vi "wifiSim.vi"(8 "error in (no error)":errorcluster, 10 "REPL":string, 11 "Server":path) -> ()   [LabVIEW 2020]
panel:
  out "concatenated string":string
  out "x .and. y?":bool
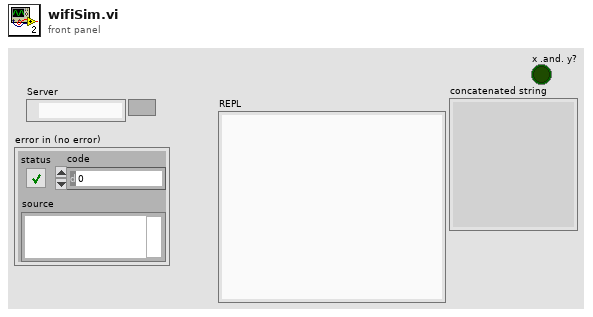
[diagram p1: front panel]
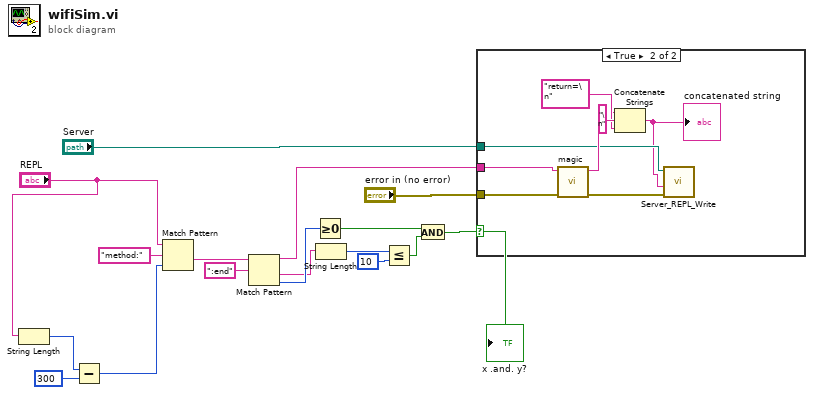
[diagram p0: block diagram]
diagram:
  n1 = String Length(string="REPL") -> (length=w3:i32)
  n2 = Subtract(x=w3, y=300) -> (x-y=w1:i32)
  n3 = Match Pattern(string="REPL", regular expression="method:" ("First"), offset (0)=w1) -> (after substring=w13:string)  [unwired: 3 out]
  n4 = Match Pattern(string=w13, regular expression=":end" ("Last")) -> (before substring=w15:string, after substring=w10:string, offset past match=w14:i32)  [unwired: 1 in, 1 out]
  n5 = Greater Or Equal To 0?(x=w14) -> (x >= 0?=w6:bool)
  n6 = String Length(string=w10) -> (length=w9:i32)
  n7 = Less Or Equal?(x=w9, y=10) -> (x <= y?=w7:bool)
  n8 = And(x=w6, y=w7) -> (x .and. y?=w5:bool)
  "x .and. y?" <- w5
  n9 = case shown="True" w5 {
    tunnel: w15 -> [_ w25]
    tunnel: "error in (no error)" -> [_ w24]
    tunnel: "Server" -> [_ w21]
    frame False {
    }
    frame True {
      n10 = call "magic.vi"("error in"=w24, "payload"=w25) -> ("error out"=w23:errorcluster, "body"=w22:string)  [unwired: 8 in]
      n11 = Concatenate Strings("\n" ("string"), w22, "return=\n" ("string")) -> (w19:string)
      "concatenated string" <- w19
      n12 = call "Server_REPL_Write.vi"("error in (no error)"=w23, "Code"=w19, "Server"=w21) -> ()  [unwired: 8 in, 1 out]
    }
  }
